vi "Demo.vi"() -> ()   [LabVIEW 2010]
panel:
  in  "stop":bool
  out "image":picture
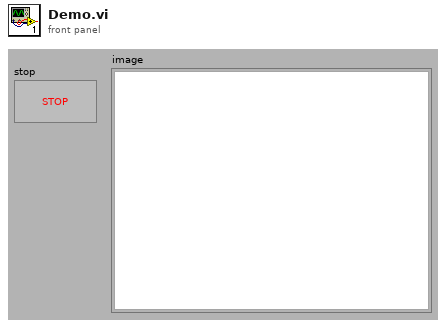
[diagram p1: front panel]
types:
  T1 = typedef "QT_Ref.ctl" = refnum<k1>
  T2 = typedef "QT_Image.ctl" = cluster{"Witdh":i32, "Height":i32, "Depth":i32, "data":u8[], "Compressed data":u8[], "Color table":u32[], "Duration":i32, "Options":i32, "Timestamp":i32, "ID":i32, "Reserved":i32, "Dialogs":u32}
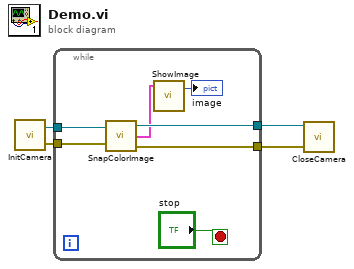
[diagram p0: block diagram]
diagram:
  n1 = call <userlib>:"InitCamera.vi"() -> ("error out"=w2:errorcluster, "QT Ref Out"=w4:T1)  [unwired: 2 in]
  n2 = while {
    tunnel: w4 -> [w11]
    tunnel: [w10] -> w3
    tunnel: w2 -> [w8]
    tunnel: [w7] -> w1
    stop <- "stop" stop-if-true
    n3 = call <userlib>:"SnapColorImage.vi"("error in (no error)"=w8, "QT Ref In"=w11) -> ("error out"=w7:errorcluster, "Image Out"=w5:T2, "QT Ref Out"=w10:T1)  [unwired: 1 in]
    n4 = call <userlib>:"ShowImage.vi"("Image"=w5) -> ("image"=→"image":picture)  [unwired: 2 in, 1 out]
  }
  n5 = call <userlib>:"CloseCamera.vi"("error in (no error)"=w1, "QT Ref In"=w3) -> ()  [unwired: 1 in, 1 out]
